vi "FA_WriteItemXML.vi"(6 "Error In":errorcluster, 7 "XML String":string, 8 "Special Type":T1) -> (0 "Error Out":errorcluster)   [LabVIEW 2014, in "FA_LocalStore.lvlib"]
doc: "Writes new Item XML to LocalStore for a given Special Type."
uses:
  FA_LocalStore.lvlib
  FA_LSSpecialTypes.ctl
  FA_LSCollections.ctl
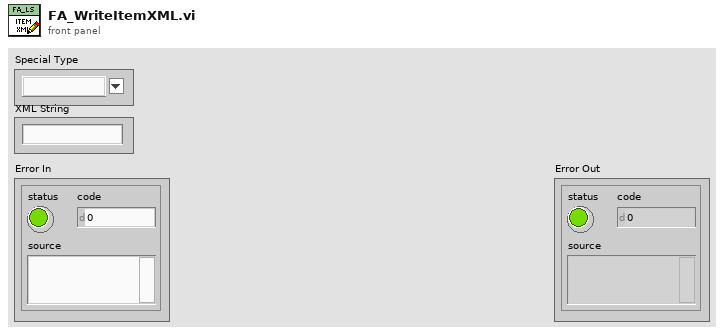
[diagram p1: front panel]
types:
  T1 = typedef "FA_LocalStore.lvlib/FA_LSSpecialTypes.ctl" = string
  T2 = typedef "FA_LocalStore.lvlib/FA_LSCollections.ctl" = enum16{"Config", "ConfigItem", "FA_eTag", "FA_PlugIn"}
  T3 = typedef "FA_LocalStore.lvlib/FA_LSRef.ctl" = cluster{"eTag INI Refnum":T4, "XML Refnum Array":refnum<file>[]}
  T4 = typedef "NI_LVConfig.lvlib/Config Data RefNum.ctl" = refnum<k1>
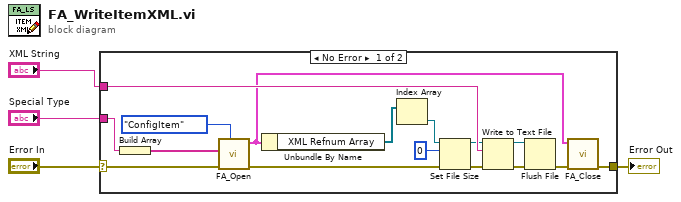
[diagram p0: block diagram]
diagram:
  n1 = case shown="No Error" "Error In" {
    selector: "Error In" -> [w7 w21]
    tunnel: [w8 w21] -> w3
    tunnel: "Special Type" -> [w11 _]
    tunnel: "XML String" -> [w20 _]
    frame No Error {
      n2 = Build Array(w11) -> (w10:T1[])
      n3 = call "FA_Open.vi"("LSCollections"=FA_LSCollections."ConfigItem", "Error In"=w7, "Special Types Array"=w10) -> ("Error Out"=w6:errorcluster, "FA_LS Ref"=w9:T3)  [unwired: 7 in]
      n4 = Unbundle By Name(w9) -> ("XML Refnum Array"=w19:refnum<file>[])
      n5 = Index Array(array=w19) -> (element=w18:refnum<file>)  [unwired: 1 in]
      n6 = Set File Size(4:w6, 6:i64 0 ("size (in bytes)"), 7:w18) -> (0:w16:errorcluster, 3:w17:refnum<file>)
      n7 = Write to Text File(file (use dialog)=w17, text=w20, error in=w16) -> (refnum out=w13:refnum<file>, error out=w14:errorcluster)  [unwired: 1 in, 1 out]
      n8 = Flush File(refnum=w13, error in=w14) -> (error out=w12:errorcluster)  [unwired: 1 out]
      n9 = call "FA_Close.vi"("Error In"=w12, "FA_LS Ref"=w9) -> ("Error Out"=w8:errorcluster)  [unwired: 9 in]
    }
    frame Error {
    }
  }
  "Error Out" <- w3
